vi "Setup AI task.vi"(8 "error in":errorcluster, 11 "DAQmx Device Name":tag) -> (0 "error out":errorcluster, 3 "task out":refnum<k21>)   [LabVIEW 2016]
uses:
  <vilib>/DAQmx/create/channels.llb/DAQmx Create Channel (AI-Voltage-Basic).vi
  <vilib>/DAQmx/configure/timing.llb/DAQmx Timing (Sample Clock).vi
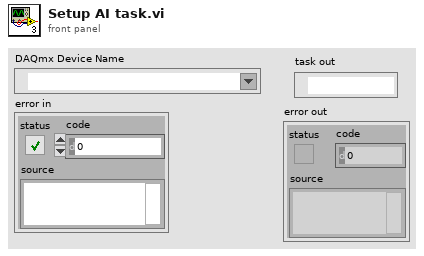
[diagram p1: front panel]
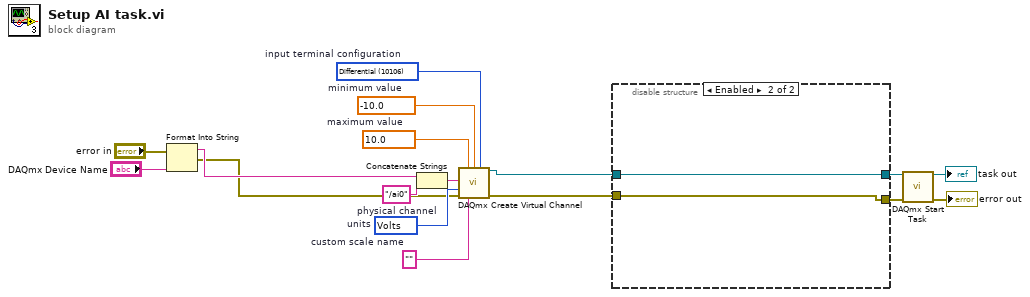
[diagram p0: block diagram]
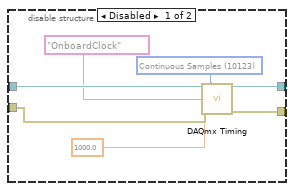
[diagram p2: hidden frame]
diagram:
  w12 = 10106 items=["default"=-1, "RSE"=10083, "NRSE"=10078, "Differential"=10106, "Pseudodifferential"=12529]  # input terminal configuration
  w13 = 10348 items=["Volts"=10348, "From Custom Scale"=10065]  # units
  w14 = ""  # custom scale name
  w15 = -10.0  # minimum value
  w16 = 10.0  # maximum value
  w17 = "/ai0"  # physical channel
  n1 = Format Into String(error in="error in", "DAQmx Device Name") -> (resulting string=w7:string, error out=w6:errorcluster)  [unwired: 2 in]
  n2 = Concatenate Strings(w7, w17) -> (w11:string)
  n3 = call-poly <vilib>:"DAQmx Create Virtual Channel.vi"("maximum value"=w16, "minimum value"=w15, "input terminal configuration"=w12, "physical channels"=w11, "units"=w13, "error in"=w6, "custom scale name"=w14) -> ("task out"=w10:refnum<k21>, "error out"=w9:errorcluster)  [unwired: 7 in]
  n4 = disable-structure shown="Enabled" {
    disable-tunnel: w10 -> [w23 w26]
    disable-tunnel: w9 -> [w22 w25]
    disable-tunnel: [w19 w25] -> w5
    disable-tunnel: [w18 w26] -> w4
    frame Disabled {
      w24 = 10123 items=["Finite Samples"=10178, "Continuous Samples"=10123, "Hardware Timed Single Point"=12522] ("sample mode")
      n5 = call-poly <vilib>:"DAQmx Timing.vi"("task/channels in"=w23, "sample mode"=w24, "rate"=1000.0, "source"=tag "OnboardClock", "error in"=w22) -> ("task out"=w18:refnum<k21>, "error out"=w19:errorcluster)  [unwired: 9 in]
    }
    frame Enabled {
    }
  }
  n6 = call <vilib>:"DAQmx Start Task.vi"("task/channels in"=w4, "error in"=w5) -> ("task out"=→"task out":refnum<k21>, "error out"=→"error out":errorcluster)  [unwired: 12 in]
